vi "createHWEvents.vi"(8 "error in (no error)":errorcluster, 11 "HWControllerEvents in":refnum<class "HWControllerEvents.lvclass">) -> (0 "error out":errorcluster, 3 "HWControllerEvents out":refnum<class "HWControllerEvents.lvclass">)   [LabVIEW 2009, in "Hardware.lvlib" / "HWControllers.lvlib" / "HWControllerEvents.lvclass"]
doc: "HWController Create Events.\n\nThese are used by the HWController and the ExperimentRunner to communicate."
uses:
  HWControllerEvents.lvclass
  HWControllerEvents.lvclass/HWControllerEvents.ctl
  HWControllers.lvlib
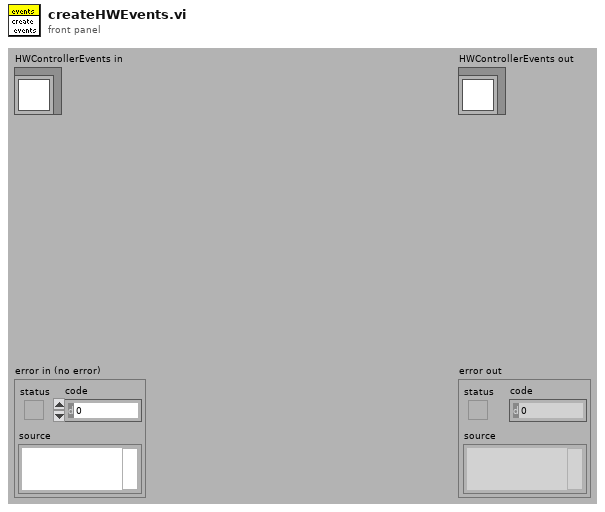
[diagram p1: front panel]
types:
  T1 = cluster{"eventId":enum16{"start", "stop", "statusInquiry", "configure", "resetError", "resourcesInquiry", "reserveResources", "initialise", "resetAllChannels", "staticUpdate", "close", "HWStatus", "error", "resourcesAvailable", "resourcesReserved", "compilerError", "compiledScript", "compilingScript", "runScript", "configureCompiledScript", "restartCompiler", "staticRfChannelUpdate"}, "data":variant}
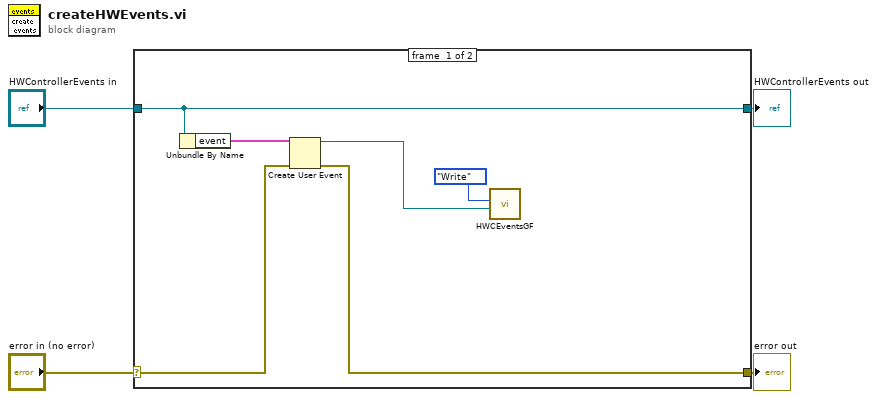
[diagram p0: block diagram]
diagram:
  n1 = case shown="No Error" "error in (no error)" {
    selector: "error in (no error)" -> [w9 w12]
    tunnel: [w8 w12] -> w3
    tunnel: [w6 w11] -> w1
    tunnel: "HWControllerEvents in" -> [w6 w11]
    frame #0 {
      n2 = Unbundle By Name(w6) -> ("event"=w10:T1)
      n3 = Create User Event(user event datatype=w10, error in=w9) -> (user event=w5:refnum<user-event>, error out=w8:errorcluster)
      n4 = call "HWCEventsGF.vi"("HWCEvent"=w5, "Action"=enum16{"Write", "Read"}."Write") -> ()  [unwired: 9 in, 1 out]
    }
    frame #1 {
    }
  }
  "error out" <- w3
  "HWControllerEvents out" <- w1
